vi "SaveControlValues.vi"(1 "sub vi path (make_current_values_default.vi)":path=path "make_current_default.vi", 2 "current vi path":path) -> ()   [LabVIEW 2018]
doc: "Run this VI if you wish to set the current values of your vi to be the default values. \n\nNote: This must be the LAST vi to execute."
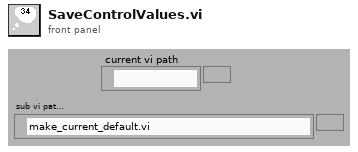
[diagram p1: front panel]
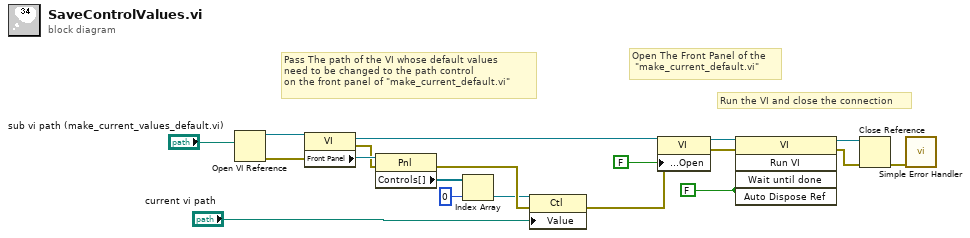
[diagram p0: block diagram]
diagram:
  w12 = FALSE ("Wait until done")
  # "Run the VI and close the connection"
  # "Pass The path of the VI whose default values\nneed to be changed to the path control\non the front panel of \"make_current_default.vi\""
  # "Open The Front Panel of the\n \"make_current_default.vi\""
  n1 = Open VI Reference(vi path="sub vi path (make_current_values_default.vi)") -> (vi reference=w5:refnum<vi>, error out=w4:errorcluster)  [unwired: 5 in]
  n2 = property class="VI"(reference=w5, error in=w4) -> (reference out=w3:refnum<vi>, error out=w7:errorcluster, "Front Panel"=w8:refnum<vi>)
  n3 = property class="Pnl"(reference=w8, error in=w7) -> (error out=w17:errorcluster, "Controls[]"=w15:refnum<vi>[])  [unwired: 1 out]
  n4 = Index Array(array=w15, index=0) -> (element=w16:refnum<vi>)
  n5 = property class="Ctl"(reference=w16, error in=w17, "Value"="current vi path") -> (error out=w18:errorcluster)  [unwired: 1 out]
  n6 = property class="VI"(reference=w3, error in=w18, "Front Panel Window:Open"=FALSE) -> (reference out=w2:refnum<vi>, error out=w1:errorcluster)
  n7 = invoke class="VI" method="Run VI"(reference=w2, error in=w1, "Wait until done"=w12, "Auto Dispose Ref"=w12) -> (reference out=w10:refnum<vi>, error out=w11:errorcluster)  [unwired: 1 in, 3 out]
  n8 = Close Reference(reference=w10, error in (no error)=w11) -> (error out=w13:errorcluster)
  n9 = call <vilib>:"Simple Error Handler.vi"("error in (no error)"=w13) -> ()  [unwired: 4 in, 5 out]
